vi "Create New Error Reported in Current One-Second Interval.vi"(1 "Error code":i32) -> (0 "Error in Current One-Second Interval":T1)   [LabVIEW 2016, in "Error Manager.lvlib"]
doc: "Blank VI with error handling."
uses:
  Error Manager.lvlib
  Error in current one-second interval (cluster).ctl
panel:
  # "Input\nInputs to the VI"
  # "Development\nControls or indicators that are useful for development or testing, but which are not outputs of the VI."
  # "Output\nOutputs of the VI"
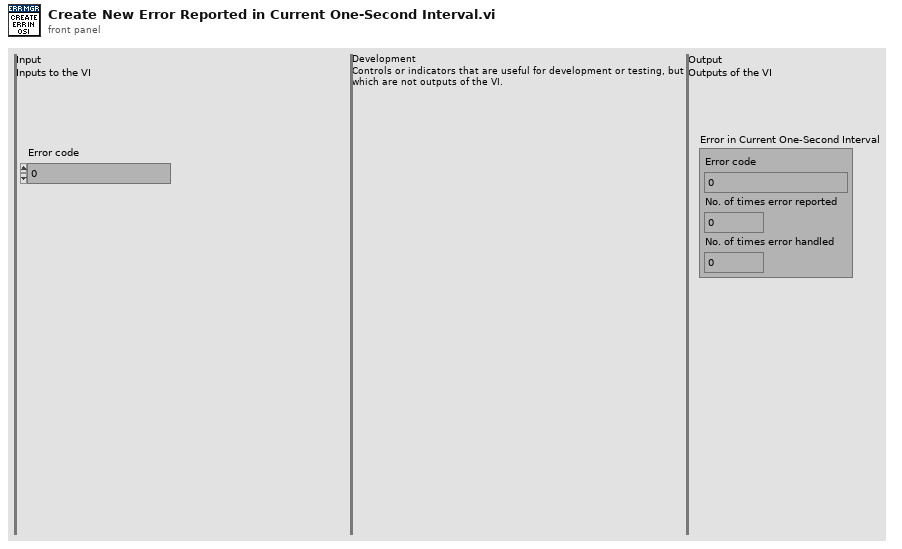
[diagram p1: front panel]
types:
  T1 = typedef "Error Manager.lvlib/Error in current one-second interval (cluster).ctl" = cluster{"Error code":i32, "No. of times error reported":u32, "No. of times error handled":u32}
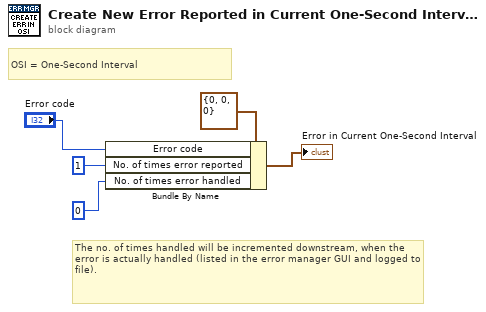
[diagram p0: block diagram]
diagram:
  # "The no. of times handled will be incremented downstream, when the error is actually handled (listed in the error manager GUI and logged to file)."
  # "OSI = One-Second Interval"
  n1 = Bundle By Name(cluster=T1 {"Error code"=0, "No. of times error reported"=0, "No. of times error handled"=0} ("Error in current one-second interval"), "Error code"="Error code", "No. of times error reported"=u32 1, "No. of times error handled"=u32 0) -> (→"Error in Current One-Second Interval":T1)
